vi "Act_cmd (SubVI).vi"(4 "W_b [rad/s]":dbl[](array[numeric]), 6 "Angles [rad]":dbl[](array[numeric]), 8 "TVA_old [rad]":dbl[](array[numeric]), 11 "TVA_cmd [rad]":dbl[](array[numeric])) -> (2 "Act315_Act225":dbl[](array[numeric]), 3 "TVA_b":dbl[](array[numeric]))   [LabVIEW 2017]
panel:
  out "roll1":dbl
  out "TVA_control_time [s]":dbl
  in  "T [s]":dbl format="%#_13g"
  out "roll_angle [rad]":dbl
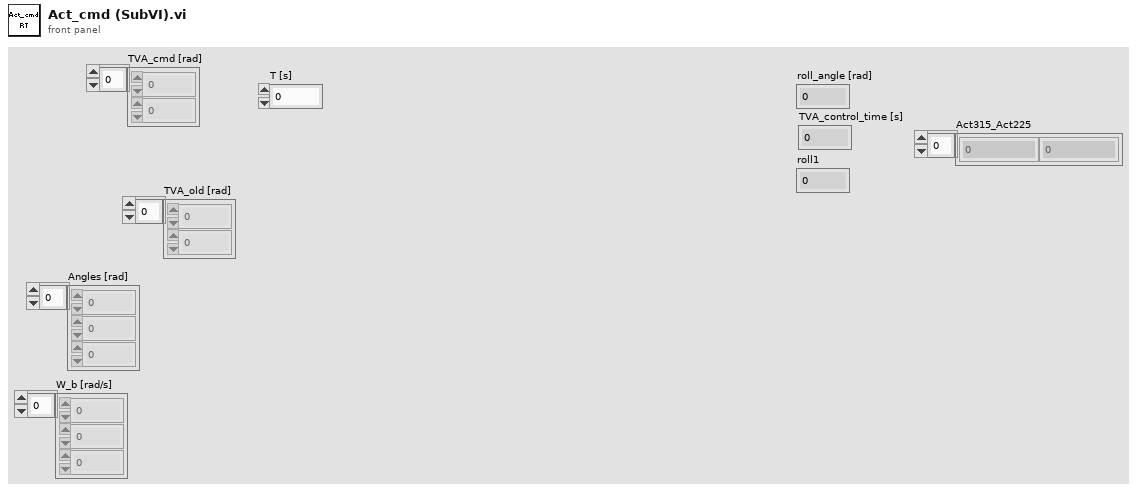
[diagram p1: front panel]
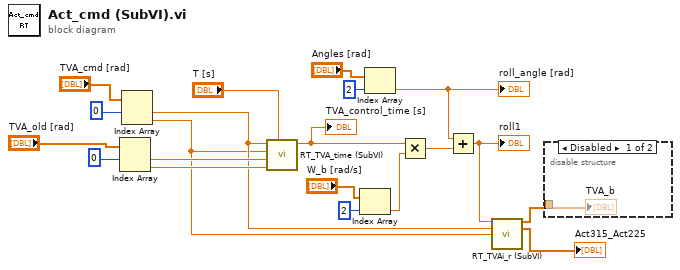
[diagram p0: block diagram]
diagram:
  n1 = Index Array(array="TVA_old [rad]", index #1=0 ("disabled index (col)")) -> (element #1=w16:dbl, element #2=w15:dbl)  [unwired: 1 in]
  n2 = Index Array(array="TVA_cmd [rad]", index #1=0 ("disabled index (col)")) -> (element #1=w14:dbl, element #2=w13:dbl)  [unwired: 1 in]
  n3 = call "RT_TVA_time (SubVI).vi"("T [s]"="T [s]", "TVA_y_old"=w15, "TVA_p_old"=w16, "TVA_y"=w13, "TVA_p"=w14) -> ("TVA_control_time [s]"=w2:dbl)  [unwired: 6 in]
  "TVA_control_time [s]" <- w2
  n4 = Index Array(array="W_b [rad/s]", index=2) -> (element=w3:dbl)
  n5 = Index Array(array="Angles [rad]", index=2) -> (element=w9:dbl)
  "roll_angle [rad]" <- w9
  n6 = Multiply(x=w2, y=w3) -> (x*y=w4:dbl)
  n7 = Add(x=w9, y=w4) -> (x+y=w10:dbl)
  "roll1" <- w10
  n8 = call "RT_TVAi_r (SubVI).vi"("roll1"=w10, "TVA_p"=w14, "TVA_y"=w13) -> ("TVA_b"=w8:dbl[], "Act315_Act225"=→"Act315_Act225":dbl[])  [unwired: 11 in]
  n9 = disable-structure shown="Disabled" {
    disable-tunnel: w8 -> [w21 _]
    frame Disabled {
      "TVA_b" <- w21
    }
    frame Enabled {
    }
  }
